vi "Data_Partitioning log.vi"() -> ()   [LabVIEW 2020]
uses:
  Global Variables/Trial_Flag.vi
  Global Variables/Trainning Done.vi
  Global Variables/Global Send To ANN.vi
panel:
  out "Array of Single":sgl[][](array[numeric])
  out "Sended frame":dbl[](array[numeric])
  out "sorted 2D array":dbl[][](array[numeric])
  out "Open File":errorcluster
  out "Pre-Partition":dbl[][](array[numeric])
  in  "stop":bool
  # "Correct"
  # "Trial n"
  # "Window n"
  # "Timestamp"
  # "Left pupil"
  # "Right pupil"
  # "Label"
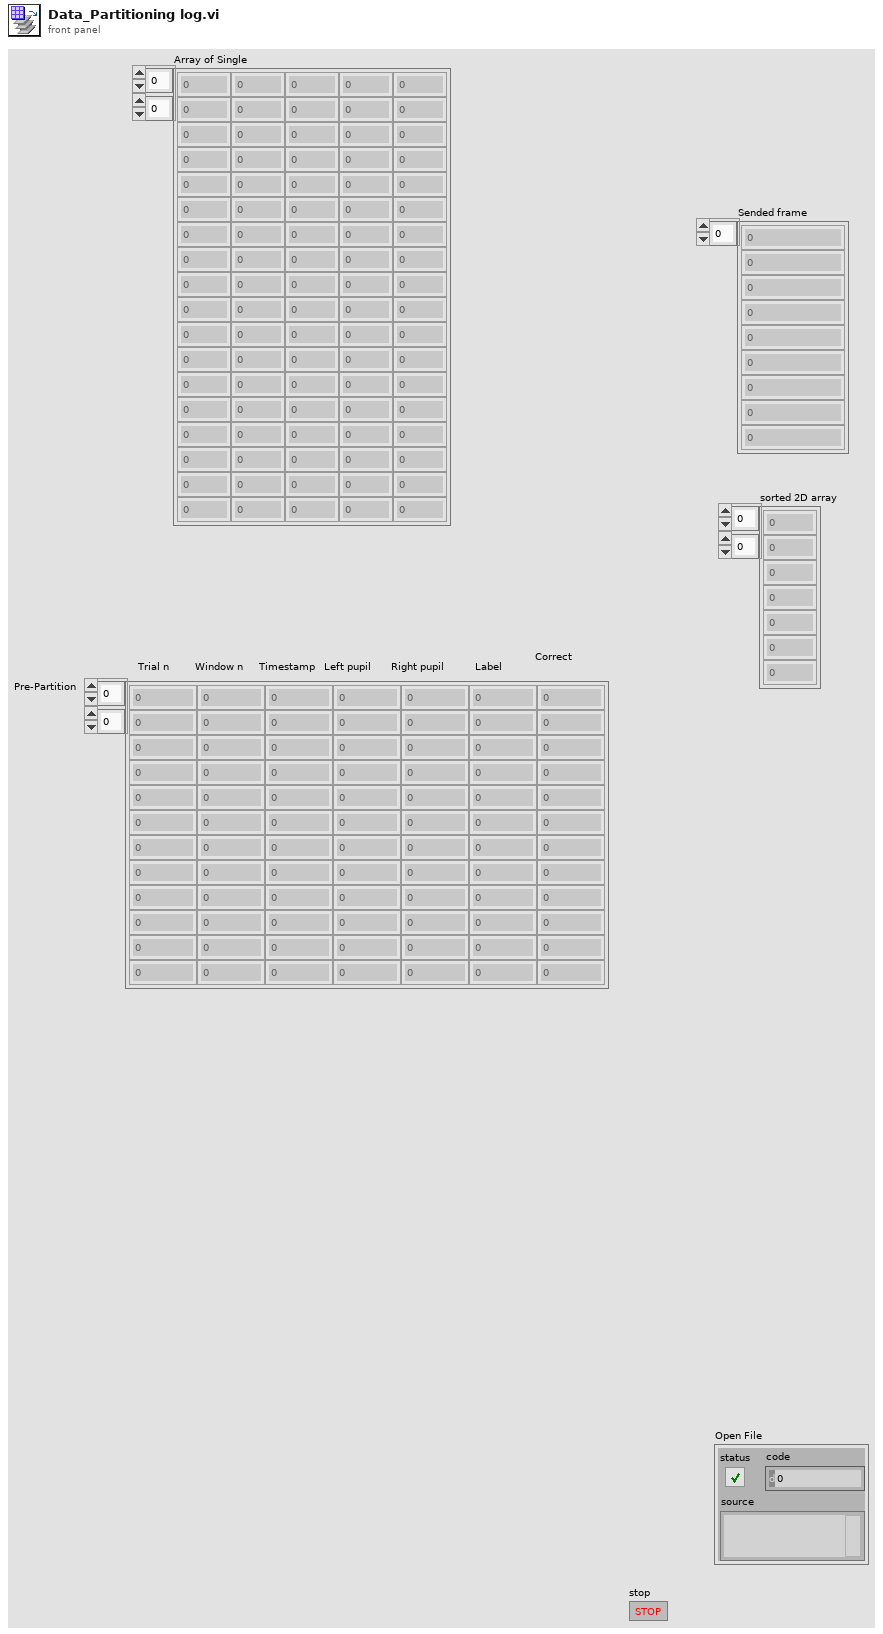
[diagram p1: front panel]
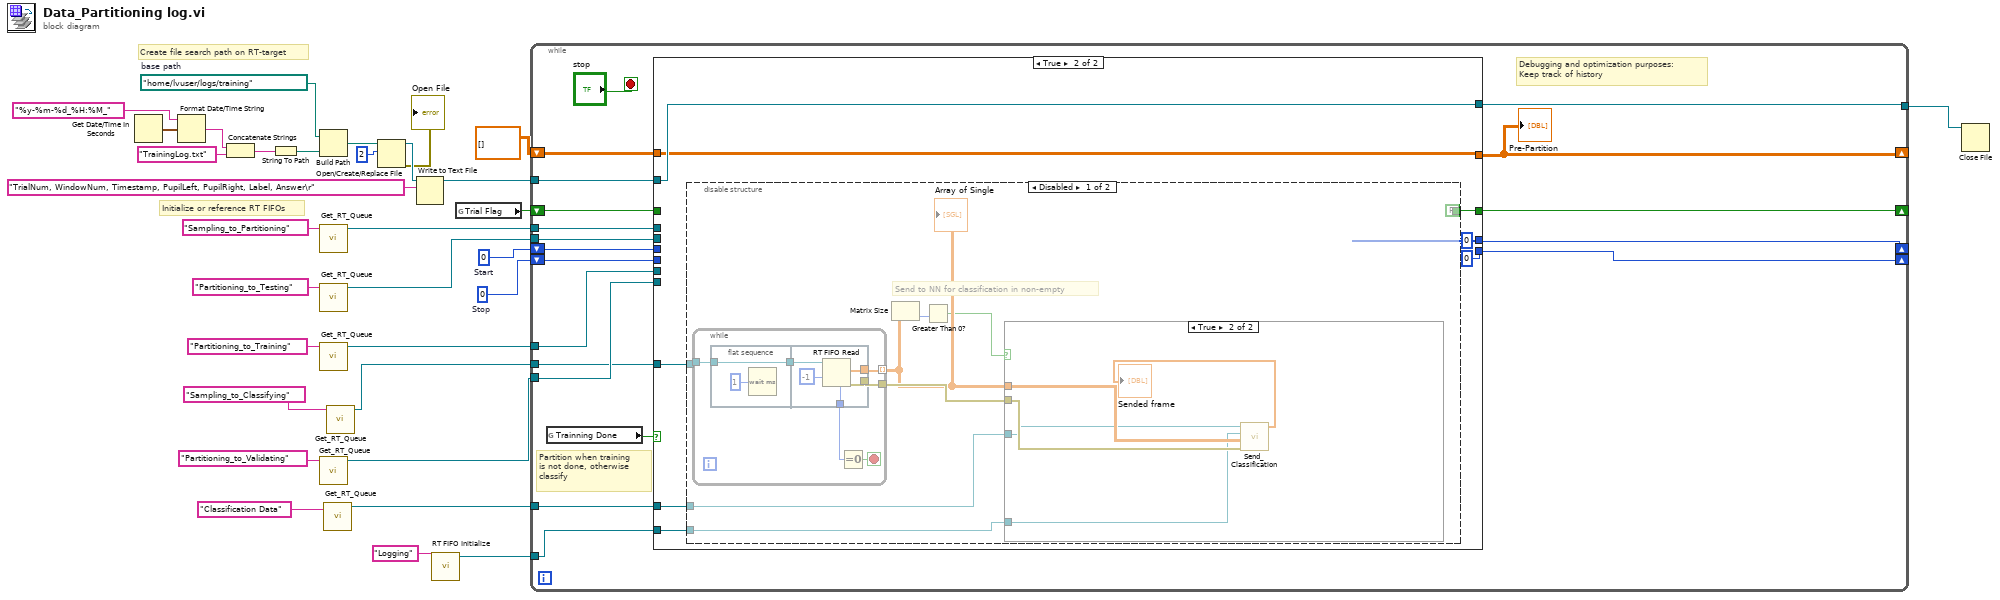
[diagram p0: block diagram]
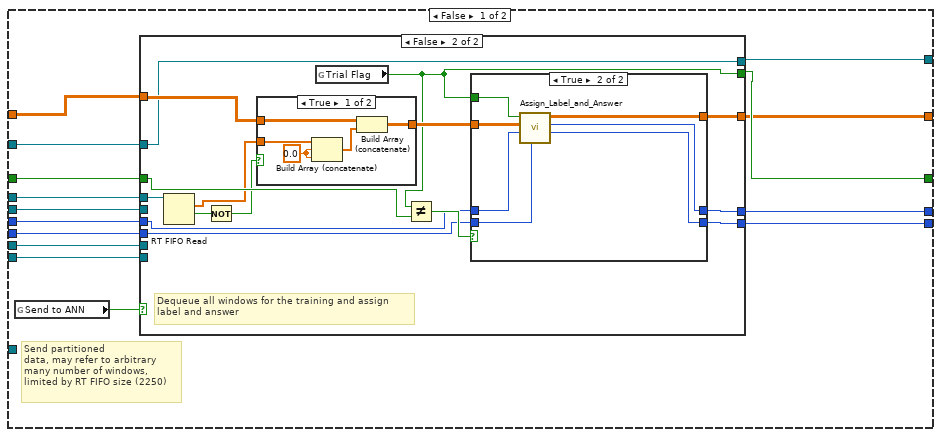
[diagram p2: hidden frame]
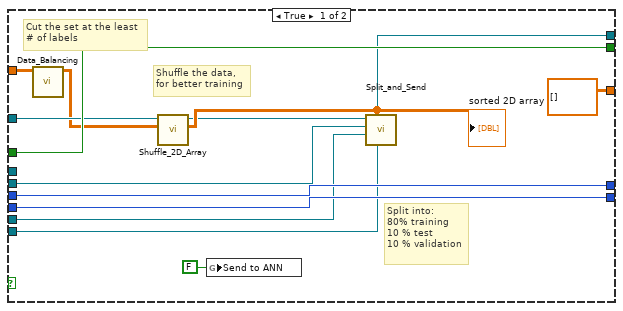
[diagram p3: hidden frame]
diagram:
  w27 = path "/home/lvuser/logs/training"  # base path
  w32 = 0  # Start
  w31 = 0  # Stop
  # "Initialize or reference RT FIFOs"
  # "Create file search path on RT-target"
  n1 = Get Date/Time In Seconds() -> (seconds since 1Jan1904=w20:timestamp)
  n2 = Format Date/Time String(time format string (%c)="%y-%m-%d_%H:%M_", seconds (now)=w20) -> (date/time string=w19:string)  [unwired: 1 in]
  n3 = Concatenate Strings(w19, "TrainingLog.txt") -> (w24:string)
  n4 = String To Path(string=w24) -> (path=w25:path)
  n5 = Build Path(base path=w27, name or relative path=w25) -> (appended path=w28:path)
  n6 = call "Get_RT_Queue.vi"("String"="Sampling_to_Partitioning") -> ("rt fifo single"=w8:refnum<k33>)  [unwired: 8 in, 2 out]
  n7 = call "Get_RT_Queue.vi"("String"="Partitioning_to_Testing") -> ("rt fifo single"=w10:refnum<k33>)  [unwired: 8 in, 2 out]
  n8 = call "Get_RT_Queue.vi"("String"="Partitioning_to_Training") -> ("rt fifo single"=w13:refnum<k33>)  [unwired: 8 in, 2 out]
  n9 = call "Get_RT_Queue.vi"("String"="Partitioning_to_Validating") -> ("rt fifo single"=w14:refnum<k33>)  [unwired: 8 in, 2 out]
  n10 = call "Get_RT_Queue.vi"("String"="Classification Data") -> ("rt fifo single"=w3:refnum<k33>)  [unwired: 8 in, 2 out]
  n11 = call "Get_RT_Queue.vi"("String"="Sampling_to_Classifying") -> ("rt fifo single"=w4:refnum<k33>)  [unwired: 8 in, 2 out]
  n12 = Open/Create/Replace File(file path (use dialog)=w28, operation (0:open)=2) -> (refnum out=w29:refnum<file>, error out=→"Open File":errorcluster)  [unwired: 4 in, 1 out]
  n13 = Write to Text File(file (use dialog)=w29, text="TrialNum, WindowNum, Timestamp, PupilLeft, PupilRight, Label, Answer\r") -> (refnum out=w22:refnum<file>)  [unwired: 2 in, 2 out]
  n14 = call "RT FIFO Initialize.vi"("name (unnamed)"="Logging") -> ("rt fifo"=w1:refnum<k33>)  [unwired: 9 in, 1 out]
  n15 = global read "Trial_Flag.vi" "Trial Flag"() -> (w30:bool)
  n16 = while {
    shift-right: [w38] -> _
    shift-left: sgl[][] [] -> [w51]
    shift-right: [w48] -> _
    shift-left: w32 -> [w46]
    shift-right: [w49] -> _
    shift-left: w31 -> [w37]
    shift-right: [w45] -> _
    shift-left: w30 -> [w47]
    tunnel: w8 -> [w44]
    tunnel: w13 -> [w43]
    tunnel: w10 -> [w42]
    tunnel: w14 -> [w41]
    tunnel: w22 -> [w40]
    tunnel: [w39] -> w17
    tunnel: w3 -> [w35]
    tunnel: w4 -> [w34]
    tunnel: w1 -> [w33]
    stop <- "stop" stop-if-true
    # "Debugging and optimization purposes: \nKeep track of history"
    # "Partition when training \nis not done, otherwise \nclassify"
    n17 = global read "Trainning Done.vi" "Trainning Done"() -> (w36:bool)
    n18 = case shown="True" w36 {
      tunnel: w51 -> [w66 w115]
      tunnel: [w65 0 ("Start out")] -> w49
      tunnel: [w64 0 ("Stop out")] -> w48
      tunnel: w47 -> [w63 _]
      tunnel: w46 -> [w62 _]
      tunnel: [w61 w117] -> w45
      tunnel: w44 -> [w60 _]
      tunnel: w43 -> [w59 _]
      tunnel: w42 -> [w58 _]
      tunnel: w41 -> [w57 _]
      tunnel: w40 -> [w56 w116]
      tunnel: [w55 w116] -> w39
      tunnel: [w54 w115] -> w38
      tunnel: w37 -> [w53 _]
      tunnel: w35 -> [_ w113]
      tunnel: w34 -> [_ w114]
      tunnel: w33 -> [_ w112]
      frame False {
        # "Send partitioned \ndata, may refer to arbitrary \nmany number of windows, \nlimited by RT FIFO size (2250)"
        n19 = global read "Global Send To ANN.vi" "Send to ANN"() -> (w52:bool)
        n20 = case shown="False" w52 {
          tunnel: w66 -> [w70 w95]
          tunnel: [w79 w93] -> w65
          tunnel: [sgl[][] [] ("Array out") w92] -> w54
          tunnel: [w78 w91] -> w64
          tunnel: w63 -> [w80 w90]
          tunnel: w62 -> [w78 w88]
          tunnel: w53 -> [w79 w87]
          tunnel: [w80 w86] -> w61
          tunnel: w60 -> [_ w85]
          tunnel: w59 -> [w77 _]
          tunnel: w58 -> [w76 _]
          tunnel: w57 -> [w75 _]
          tunnel: w56 -> [w73 w83]
          tunnel: [w71 w83] -> w55
          frame True {
            # "Split into: \n80% training \n10 % test \n10 % validation"
            # "Shuffle the data, \nfor better training"
            # "Cut the set at the least \n# of labels"
            n21 = call "Data_Balancing.vi"("Array in"=w70) -> ("Array out"=w69:sgl[][])  [unwired: 10 in]
            n22 = call "Shuffle_2D_Array.vi"("Array"=w69, "Byte Stream File in"=w73) -> ("sorted 2D array"=w74:dbl[][], "Byte Stream File out"=w72:refnum<file>)  [unwired: 8 in]
            "sorted 2D array" <- w74
            n23 = global write "Global Send To ANN.vi" "Send to ANN"(FALSE ("Send to ANN")) -> ()
            n24 = call "Split_and_Send.vi"("rt fifo"=w75, "sorted 2D array"=w74, "rt fifo 3"=w77, "rt fifo 2"=w76, "Byte Stream File in"=w72) -> ("Byte Stream File out"=w71:refnum<file>)  [unwired: 6 in]
          }
          frame False {
            # "Dequeue all windows for the training and assign \nlabel and answer"
            n25 = RT FIFO Read(0:w85) -> (9:w84:sgl[], 10:w82:bool)  [unwired: 3 in, 3 out]
            n26 = Not(x=w82) -> (.not. x?=w81:bool)
            n27 = case shown="True" w81 {
              tunnel: w95 -> [w109 w111]
              tunnel: [w110 w111] -> w94
              tunnel: w84 -> [w108 _]
              frame True {
                w107 = sgl 0.0
                n28 = Build Array (concatenate)(w108, w107, w107) -> (w106:sgl[])
                n29 = Build Array (concatenate)(w109, w106) -> (w110:sgl[][])
              }
              frame False {
              }
            }
            n30 = global read "Trial_Flag.vi" "Trial Flag"() -> (w86:bool)
            n31 = Not Equal?(x=w86, y=w90) -> (x != y?=w89:bool)
            n32 = case shown="True" w89 {
              tunnel: w94 -> [w98 w105]
              tunnel: w88 -> [w97 w101]
              tunnel: w87 -> [w96 w103]
              tunnel: [w96 w102] -> w93
              tunnel: [w98 w104] -> w92
              tunnel: [w97 w100] -> w91
              tunnel: w86 -> [_ w99]
              frame False {
              }
              frame True {
                n33 = call "Assign_Label_and_Answer.vi"("Start in"=w103, "Stop in"=w101, "Array in"=w105, "Trial Flag"=w99) -> ("Start out"=w102:i32, "Stop out"=w100:i32, "Array out"=w104:sgl[][])  [unwired: 5 in]
              }
            }
          }
        }
      }
      frame True {
        n34 = disable-structure shown="Disabled" {
          disable-tunnel: [FALSE ("Trial Flag") _] -> w117
          disable-tunnel: w114 -> [w122 _]
          disable-tunnel: w113 -> [w121 _]
          disable-tunnel: w112 -> [w120 _]
          frame Disabled {
            # "Send to NN for classification in non-empty"
            n35 = while {
              tunnel: w122 -> [w138]
              tunnel: [w136] -> w125 mode=indexing
              tunnel: [w135] -> w126
              stop <- w134 stop-if-true
              n36 = flat-sequence {
                tunnel: w138 -> [w140]
                tunnel: [w140] -> w133
                tunnel: [w144] -> w137
                tunnel: [w143] -> w136
                tunnel: [w142] -> w135
                tunnel: w133 -> [w145]
                frame #0 {
                  n37 = Wait (ms)(milliseconds to wait=u32 1) -> ()  [unwired: 1 out]
                }
                frame #1 {
                  n38 = RT FIFO Read(0:w145, 2:-1 ("timeout in ms (0)")) -> (7:w144:u32, 9:w143:sgl[], 11:w142:errorcluster)  [unwired: 2 in, 2 out]
                }
              }
              n39 = Equal To 0?(x=w137) -> (x = 0?=w134:bool)
            }
            "Array of Single" <- w125
            n40 = Matrix Size(0:w125) -> (2:w123:i32)  [unwired: 1 out]
            n41 = Greater Than 0?(x=w123) -> (x > 0?=w124:bool)
            n42 = case shown="True" w124 {
              tunnel: w125 -> [_ w132]
              tunnel: w126 -> [_ w131]
              tunnel: w121 -> [_ w130]
              tunnel: w120 -> [_ w129]
              frame False {
              }
              frame True {
                n43 = call "Send_Classification.vi"("error in (no error)"=w131, "Window"=w132, "logging FIFO"=w129, "Classification FIFO"=w130) -> ("Sended frame"=→"Sended frame":dbl[])  [unwired: 7 in]
              }
            }
          }
          frame Enabled {
          }
        }
      }
    }
    "Pre-Partition" <- w38
  }
  n44 = Close File(refnum=w17) -> ()  [unwired: 1 in, 2 out]
